vi "Rename Class Input and Output.vi"(8 "error in (no error)":errorcluster, 11 "QControl Creation in":refnum<class "QControl Creation.lvclass">) -> (0 "error out":errorcluster, 3 "QControl Creation (dup)":refnum<class "QControl Creation.lvclass">)   [LabVIEW 2015, in "QControl Creation.lvclass"]
doc: "<b> </b> <b> </b>\n©2016 Q Software Innovations, LLC (QSI)\nwritten by Quentin Alldredge\nproduced in LabVIEW 2015\n\nsupport@qsoftwareinnovations.com\nwww.qsoftwareinnovations.com\n\nAll rights reserved.\n\nRedistribution and use in source and binary forms, with or without modification, are permitted provided that the following conditions are met:\n\n * Redistributions of source code must retain the above copyright notice, this list of conditions and the following disclaimer.\n * Redistributions in binary form must reproduce the above copyright notice, this list of conditions and the following disclaimer in the documentation and/or other materials provided with the distribution.\n * Neither the name of Q Software Innovations, LLC. nor the names of its contributors may be used to endorse or promote products derived from this software without specific prior written permission.\n\nTHIS SOFTWARE IS PROVIDED BY THE COPYRIGHT HOLDERS AND CONTRIBUTORS \"AS IS\" AND ANY EXPRESS OR IMPLIED WARRANTIES, INCLUDING, BUT NOT LIMITED TO, THE IMPLIED WARRANTIES OF MERCHANTABILITY AND FITNESS FOR A PARTICULAR PURPOSE ARE DISCLAIMED. IN NO EVENT SHALL THE COPYRIGHT OWNER OR CONTRIBUTORS BE LIABLE FOR ANY DIRECT, INDIRECT, INCIDENTAL, SPECIAL, EXEMPLARY, OR CONSEQUENTIAL DAMAGES (INCLUDING, BUT NOT LIMITED TO, PROCUREMENT OF SUBSTITUTE GOODS OR SERVICES; LOSS OF USE, DATA, OR PROFITS; OR BUSINESS INTERRUPTION) HOWEVER CAUSED AND ON ANY THEORY OF LIABILITY, WHETHER IN CONTRACT, STRICT LIABILITY, OR TORT (INCLUDING NEGLIGENCE OR OTHERWISE) ARISING IN ANY WAY OUT OF THE USE OF THIS SOFTWARE, EVEN IF ADVISED OF THE POSSIBILITY OF SUCH DAMAGE."
uses:
  QControl Creation.lvclass
  QControl Creation.lvclass/QControl Creation.ctl
  New QControl Info/New QControl Info.lvclass/New QControl Info.ctl
  New QControl Info/Read New Class Path.vi
  New QControl Info/Read Localized Name.vi
  <vilib>/Utility/error.llb/Error Cluster From Error Code.vi
  <vilib>/ErrorRing/Error Ring.xnode
  New QControl Info/New QControl Info.lvclass
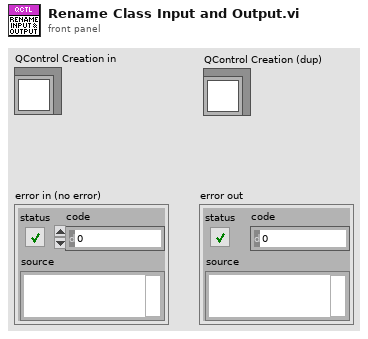
[diagram p1: front panel]
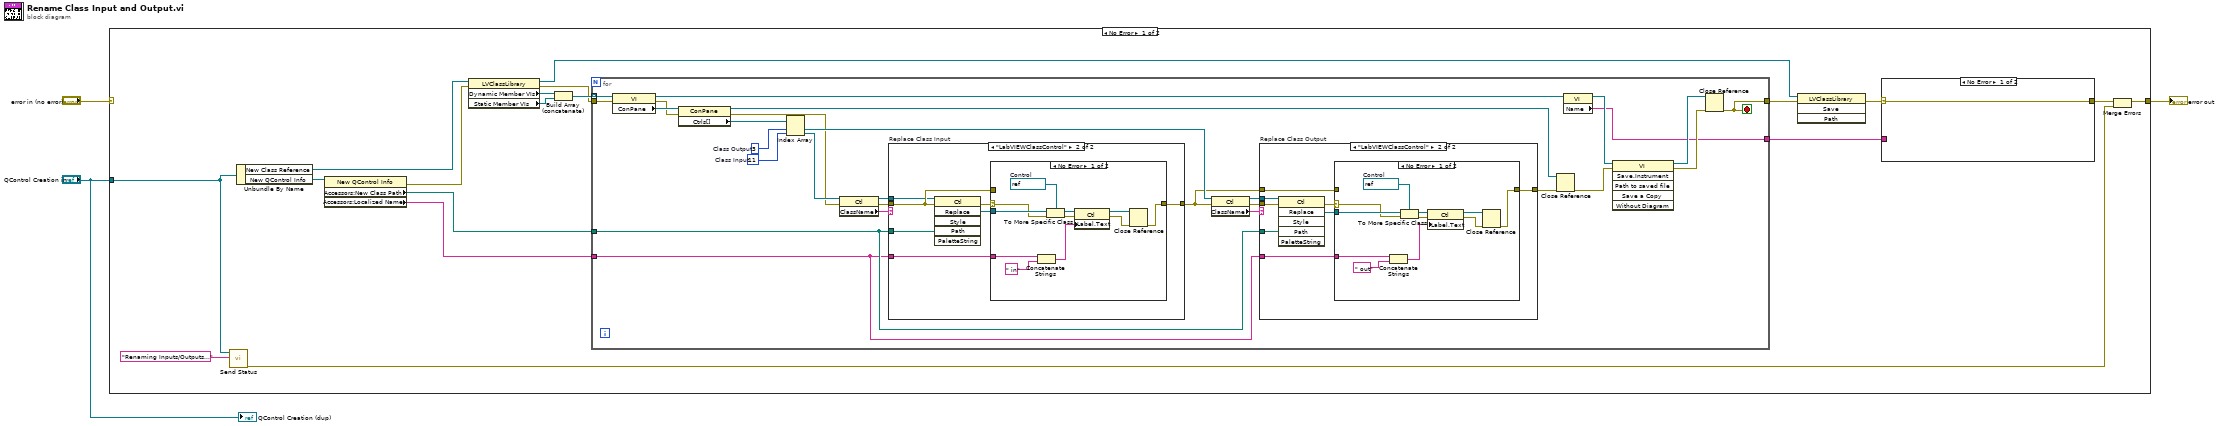
[diagram p0: block diagram]
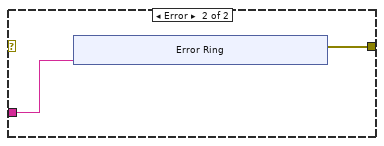
[diagram p2: hidden frame]
diagram:
  n1 = case shown="No Error" "error in (no error)" {
    selector: "error in (no error)" -> [_ w101]
    tunnel: [w11 w101] -> w3
    tunnel: "QControl Creation in" -> [w12 _]
    frame No Error {
      n2 = call "Send Status.vi"("Status"="Renaming Inputs/Outputs..." ("Value"), "QControl Creation in"=w12) -> ("error out (dup)"=w10:errorcluster)  [unwired: 8 in, 1 out]
      n3 = Unbundle By Name(w12) -> ("New Class Reference"=w17:refnum<vi>, "New QControl Info"=w18:refnum<data-value>)
      n4 = property class="New QControl Info"(reference=w18) -> (error out=w4:errorcluster, "Accessors:New Class Path"=w6:path, "Accessors:Localized Name"=w5:string)  [unwired: 1 in, 1 out]
      n5 = property class="LVClassLibrary"(reference=w17, error in=w4) -> (reference out=w15:refnum<vi>, error out=w14:errorcluster, "Dynamic Member VIs"=w19:refnum<vi>[], "Static Member VIs"=w20:refnum<vi>[])
      n6 = Build Array (concatenate)(w19, w20) -> (w21:refnum<vi>[])
      n7 = for {
        tunnel: w21 -> [w59] mode=indexing
        tunnel: w6 -> [w53]
        tunnel: w5 -> [w35]
        tunnel: w14 -> [w51]
        tunnel: [w34] -> w16
        tunnel: [w32] -> w9
        stop <- w34 stop-if-true
        w56 = 3  # Class Output
        w55 = 11  # Class Input
        n8 = property class="VI"(reference=w59, error in=w51) -> (reference out=w48:refnum<vi>, error out=w52:errorcluster, "ConPane"=w58:refnum<vi>)
        n9 = property class="ConPane"(reference=w58, error in=w52) -> (reference out=w50:refnum<vi>, error out=w37:errorcluster, "Ctrls[]"=w57:refnum<vi>[])
        n10 = Index Array(array=w57, index #1=w56, index #2=w55) -> (element #1=w42:refnum<vi>, element #2=w54:refnum<vi>)
        n11 = property class="Ctl"(reference=w54, error in=w37) -> (reference out=w44:refnum<vi>, error out=w36:errorcluster, "ClassName"=w43:string)
        n12 = case "Replace Class Input" shown="\"LabVIEWClassControl\"" w43 {
          tunnel: w53 -> [_ w67]
          tunnel: w35 -> [_ w65]
          tunnel: w36 -> [w60 w63]
          tunnel: [w60 w62] -> w40
          tunnel: w44 -> [_ w61]
          frame Default {
          }
          frame "LabVIEWClassControl" {
            n13 = invoke class="Ctl" method="Replace"(reference=w61, error in=w63, "Path"=w67) -> (error out=w64:errorcluster, "Replace"=w66:refnum<vi>)  [unwired: 3 in, 4 out]
            n14 = case shown="No Error" w64 {
              selector: w64 -> [w73 _]
              tunnel: w66 -> [w78 _]
              tunnel: w65 -> [w68 _]
              tunnel: [w74 w79] -> w62
              tunnel: w63 -> [_ w79]
              frame No Error {
                w71 = refnum<vi> refnum  # Control
                n15 = Concatenate Strings(w68, " in" ("string")) -> (w69:string)
                n16 = To More Specific Class(target class=w71, reference=w78, error in=w73) -> (specific class reference=w77:refnum<vi>, error out=w72:errorcluster)
                n17 = property class="Ctl"(reference=w77, error in=w72, "Label.Text"=w69) -> (reference out=w76:refnum<vi>, error out=w75:errorcluster)
                n18 = Close Reference(reference=w76, error in (no error)=w75) -> (error out=w74:errorcluster)
              }
              frame Error {
              }
            }
          }
        }
        n19 = property class="Ctl"(reference=w42, error in=w40) -> (reference out=w41:refnum<vi>, error out=w39:errorcluster, "ClassName"=w38:string)
        n20 = case "Replace Class Output" shown="\"LabVIEWClassControl\"" w38 {
          tunnel: w53 -> [_ w88]
          tunnel: w35 -> [_ w86]
          tunnel: [w80 w84] -> w49
          tunnel: w41 -> [_ w83]
          tunnel: w40 -> [w80 w82]
          tunnel: w39 -> [_ w81]
          frame Default {
          }
          frame "LabVIEWClassControl" {
            n21 = invoke class="Ctl" method="Replace"(reference=w83, error in=w81, "Path"=w88) -> (error out=w85:errorcluster, "Replace"=w87:refnum<vi>)  [unwired: 3 in, 4 out]
            n22 = case shown="No Error" w85 {
              selector: w85 -> [w94 _]
              tunnel: w87 -> [w98 _]
              tunnel: w86 -> [w90 _]
              tunnel: [w93 w100] -> w84
              tunnel: w82 -> [_ w100]
              frame No Error {
                w92 = refnum<vi> refnum  # Control
                n23 = Concatenate Strings(w90, " out" ("string")) -> (w89:string)
                n24 = To More Specific Class(target class=w92, reference=w98, error in=w94) -> (specific class reference=w99:refnum<vi>, error out=w96:errorcluster)
                n25 = property class="Ctl"(reference=w99, error in=w96, "Label.Text"=w89) -> (reference out=w97:refnum<vi>, error out=w95:errorcluster)
                n26 = Close Reference(reference=w97, error in (no error)=w95) -> (error out=w93:errorcluster)
              }
              frame Error {
              }
            }
          }
        }
        n27 = Close Reference(reference=w50, error in (no error)=w49) -> (error out=w46:errorcluster)
        n28 = property class="VI"(reference=w48) -> (reference out=w33:refnum<vi>, "Name"=w32:string)  [unwired: 1 in, 1 out]
        n29 = invoke class="VI" method="Save.Instrument"(reference=w33, error in=w46) -> (reference out=w47:refnum<vi>, error out=w45:errorcluster)  [unwired: 4 in, 4 out]
        n30 = Close Reference(reference=w47, error in (no error)=w45) -> (error out=w34:errorcluster)
      }
      n31 = invoke class="LVClassLibrary" method="Save"(reference=w15, error in=w16) -> (error out=w8:errorcluster)  [unwired: 2 in, 3 out]
      n32 = case shown="No Error" w8 {
        selector: w8 -> [w22 _]
        tunnel: w9 -> [_ w24]
        tunnel: [w22 w23] -> w7
        frame No Error {
        }
        frame Error {
          n33 = xnode "Error Ring"("parameter 0"=w24) -> ("error out"=w23:errorcluster)
        }
      }
      n34 = Merge Errors(w7, w10) -> (w11:errorcluster)
    }
    frame Error {
    }
  }
  "error out" <- w3
  "QControl Creation (dup)" <- "QControl Creation in"
